vi "TDMS - File Viewer.vi"(4 "error in (no error)":errorcluster, 7 "file path":path) -> (0 "error out":errorcluster, 3 "file path out":path)   [LabVIEW 2017]
doc: "<B>Copyright:</B> (c) 2017 National Instruments. All rights reserved.\n\nOpens the .tdms file specified in the <B>file path</B> input and presents the file data in the TDMS File Viewer dialog box."
uses:
  <vilib>/Utility/tdmsutil.llb/fileViewerConfigData.ctl
  <vilib>/Utility/error.llb/DialogType.ctl
  <vilib>/event_ctls.llb/sizeaction.ctl
  <vilib>/event_ctls.llb/panelstate.ctl
  <vilib>/Utility/tdmsutil.llb/TDMSFileViewerLocalizedText.vi
  Instance           1 26Saved   TDMS - File Viewer .vi
panel:
  out "LastXScaleFormat":u8
  out "TotalCount":u64
  out "Temp Configuration":T1
  in  "LastTopLeftValue":u64
  out "Resize?":bool
  in  "Help":bool
  in  "Status":string
  in  "Quit":bool
  in  "Settings...":bool
  in  "Properties / Values / Graph":T2(tab)
  in  "Properties":i32(listbox)
  in  "Go To":bool
  in  "Scrollbar":u64(c297)
  in  "Raw data values":i32(listbox)
  out "Waveform Graph":waveform(dbl)[](graph)
  in  "File contents":string(tree)
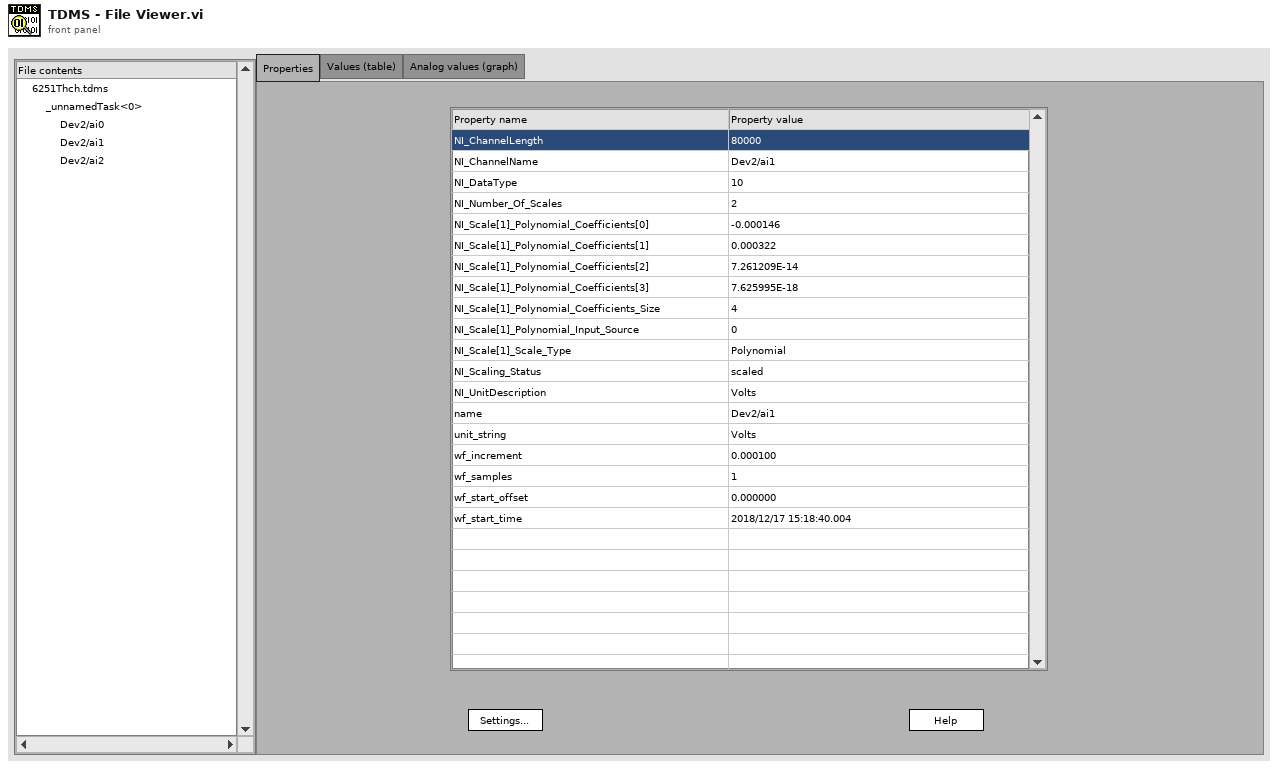
[diagram p1: front panel]
types:
  T1 = typedef "fileViewerConfigData.ctl" = cluster{"Show all (table)":bool, "Show all (graph)":bool, "limit (table)":u64, "limit (graph)":u64, "no show":bool, "start (table)":u64, "start (graph)":u64}
  T2 = enum32{"Properties", "Values (table)", "Analog values (graph)"}
  T3 = enum16{"open", "open or create", "create or replace", "create", "open (read-only)"}
  T4 = cluster{"Tree":refnum<vi>, "Tab Control":refnum<vi>, "property list":refnum<vi>, "raw data list":refnum<vi>, "Waveform Graph":refnum<vi>, "Ok":refnum<vi>, "Ok 2":refnum<vi>, "Ok 3":refnum<vi>, "Ok 4":refnum<vi>, "Scrollbar":refnum<vi>, "Ok 5":refnum<vi>, "TopLeftValue":refnum<vi>, "TotalCount":refnum<vi>}
  T5 = typedef "panelstate.ctl" = enum32{"Standard", "Minimized", "Maximized"}
  T6 = typedef "sizeaction.ctl" = enum32{"Minimized", "Maximized", "Resized"}
  T7 = cluster{"Shift":bool, "Ctrl":bool, "Alt":bool, "Cmd":bool, "Opt":bool}
  T8 = typedef "LVRectTypeDef.ctl" = cluster{"Left":i16, "Top":i16, "Right":i16, "Bottom":i16}
  T9 = typedef "LVRowAndColumnUnsignedTypeDef.ctl" = cluster{"Row":u32, "Column":u32}
  T10 = typedef "DialogType.ctl" = u16
  T11 = typedef "eventvkey.ctl" = enum16{"ASCII", "Enter", "Return", "Shift", "Ctrl", "Alt", "Cmd", "Opt", "Caps", "NumLock", "Clear", "Break", "Up", "Down", "Left", "Right", "Insert", "Delete", "Home", "End", "PageUp", "PageDown", "Escape", "Help", "Pause", "ScrollLock", "F1", "F2", "F3", "F4", "F5", "F6", "F7", "F8", "F9", "F10", "F11", "F12", "F13", "F14", "F15", "F16", "F17", "F18", "F19", "F20", "F21", "F22", "F23", "F24", "Play", "VolumeUp", "VolumeDown", "Mute", "Two Byte Char"}
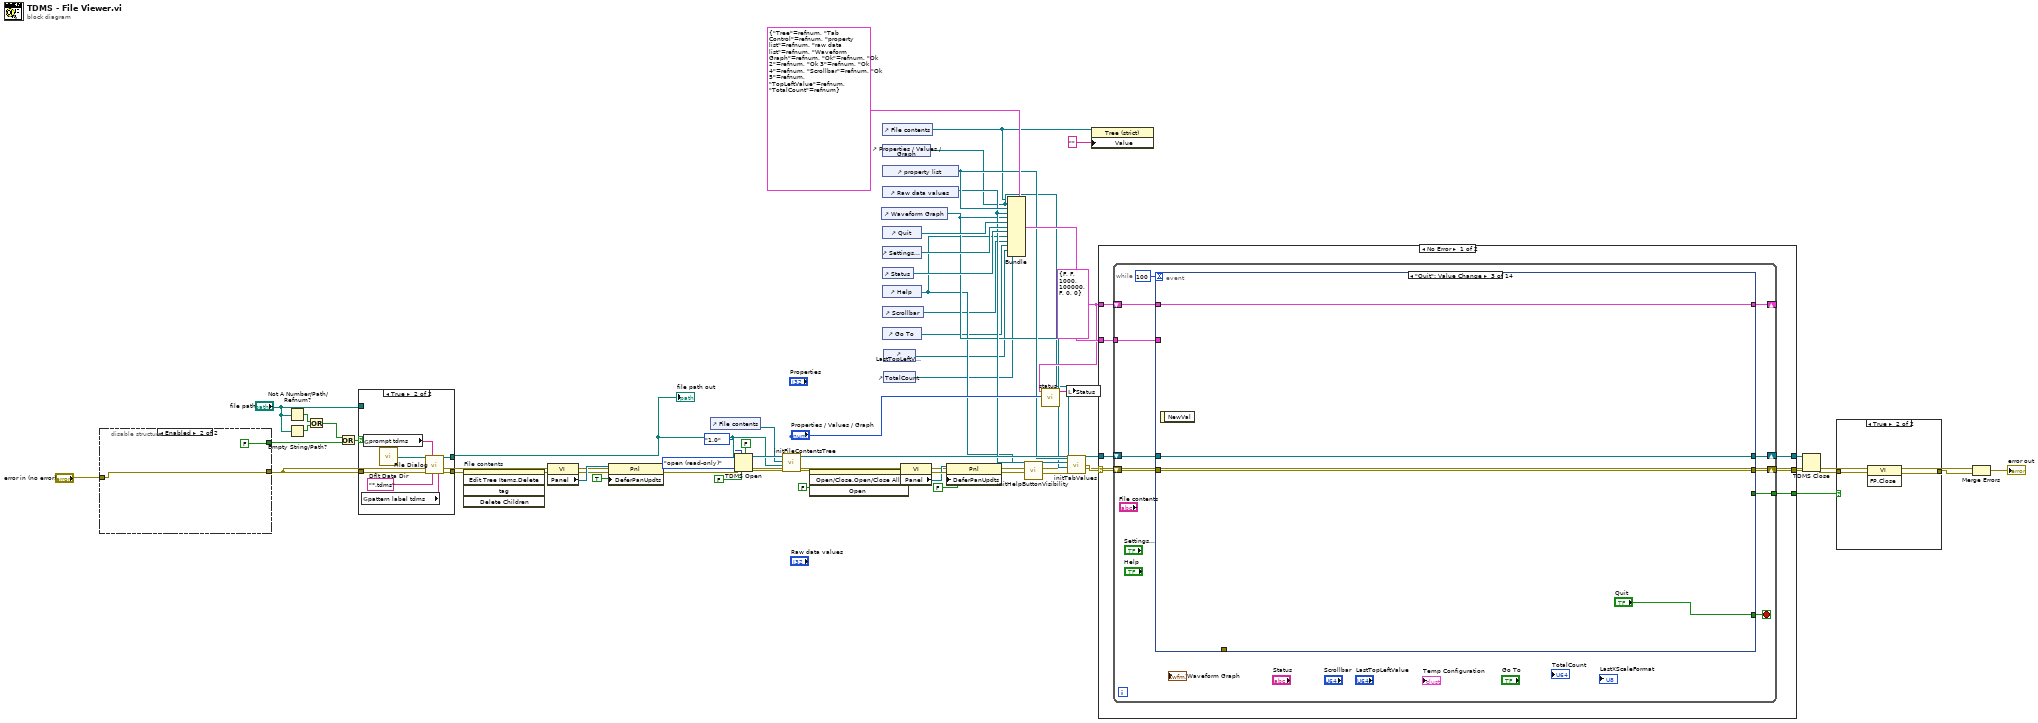
[diagram p0: block diagram]
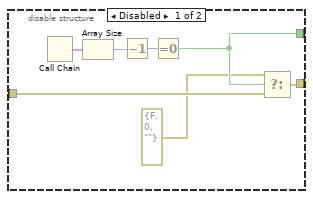
[diagram p2: hidden frame]
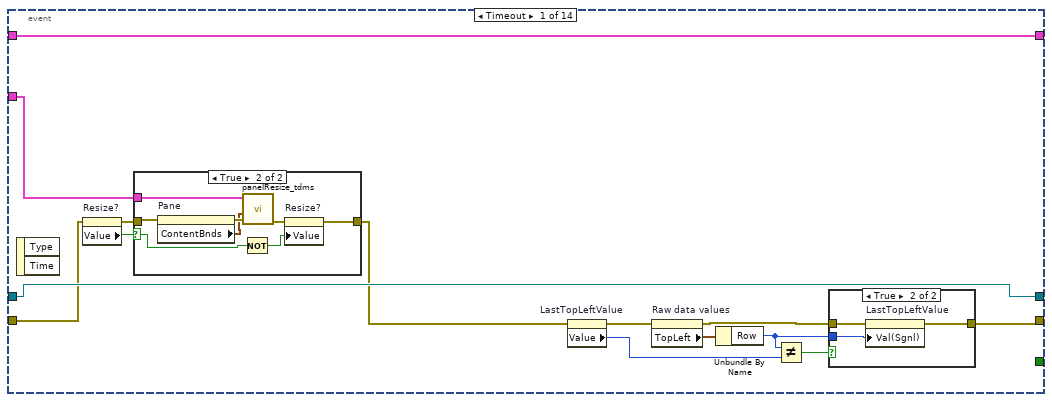
[diagram p4: hidden frame]
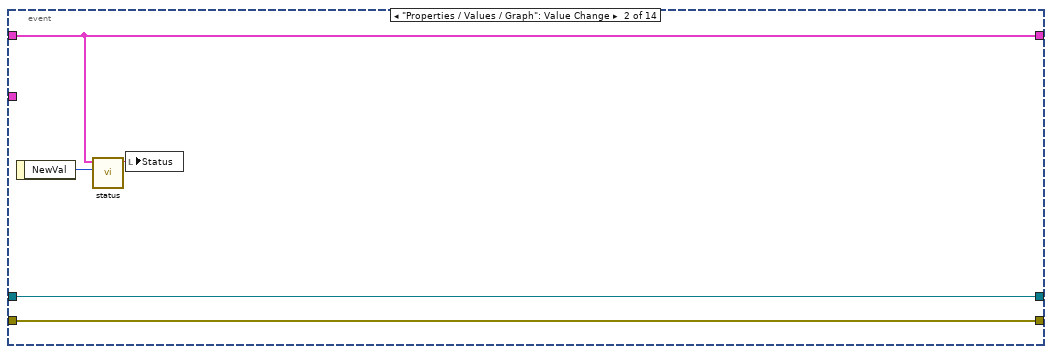
[diagram p7: hidden frame]
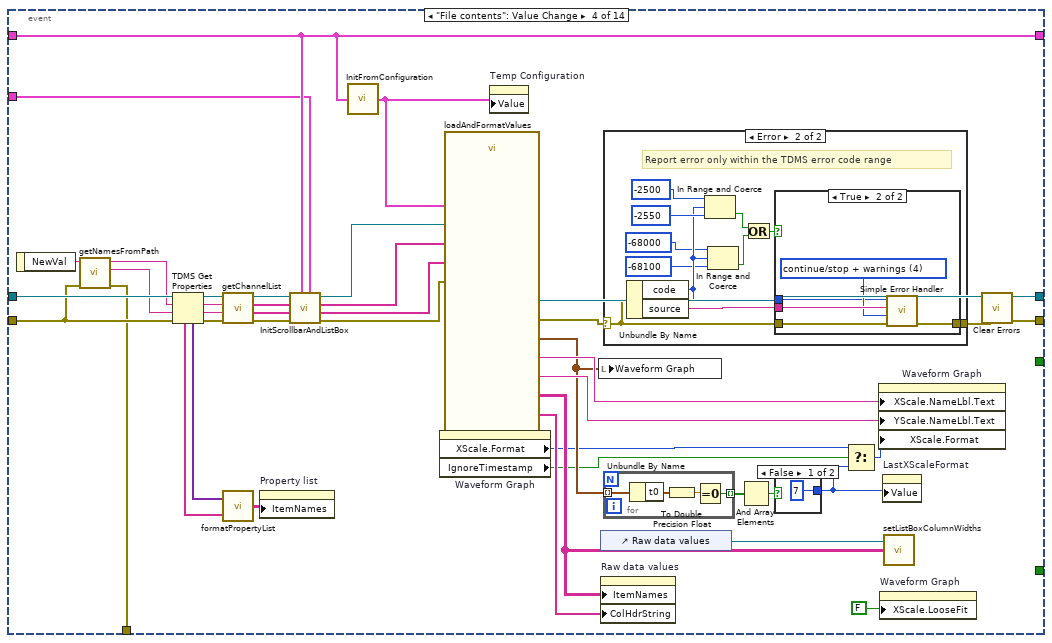
[diagram p8: hidden frame]
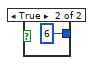
[diagram p9: hidden frame]
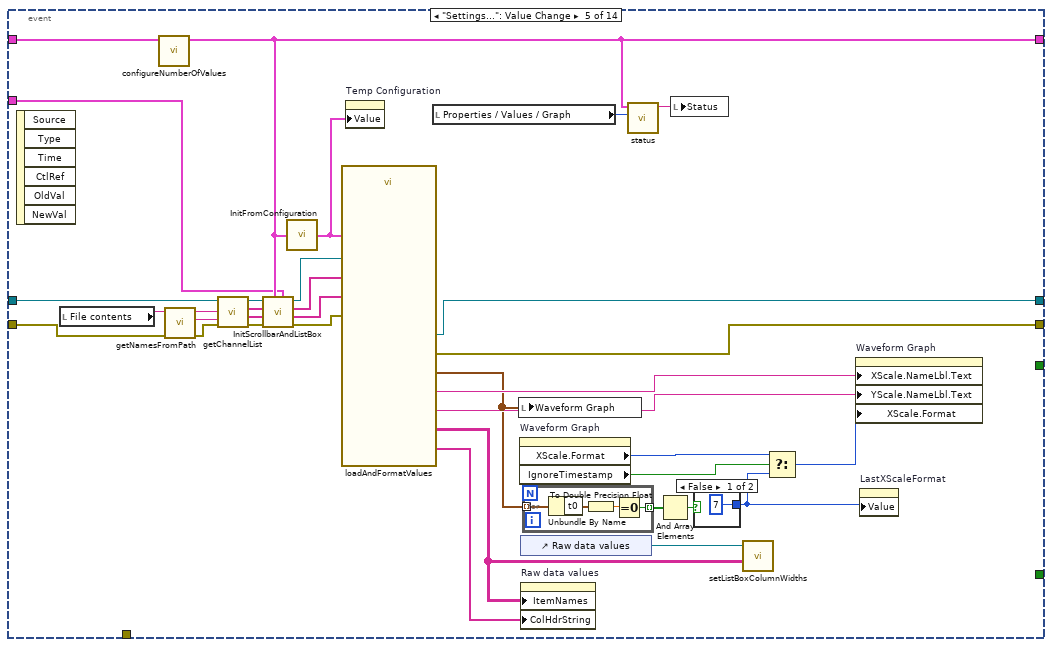
[diagram p12: hidden frame]
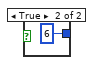
[diagram p13: hidden frame]
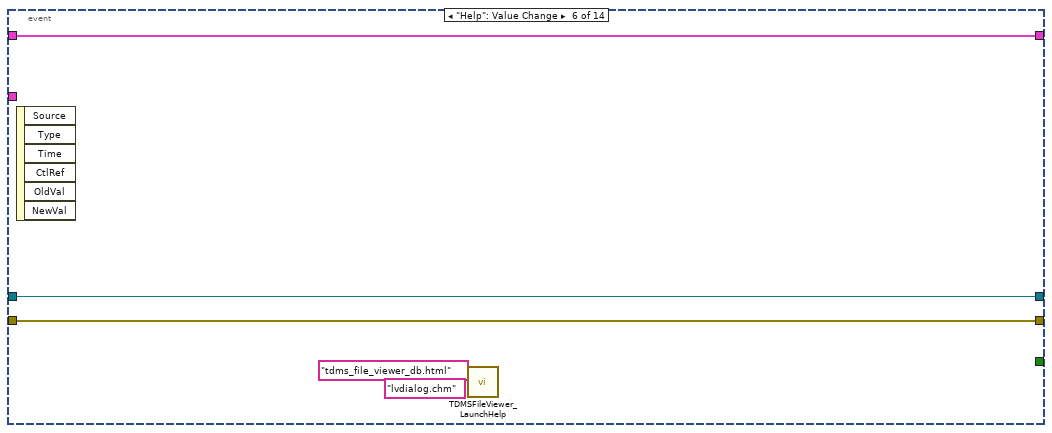
[diagram p14: hidden frame]
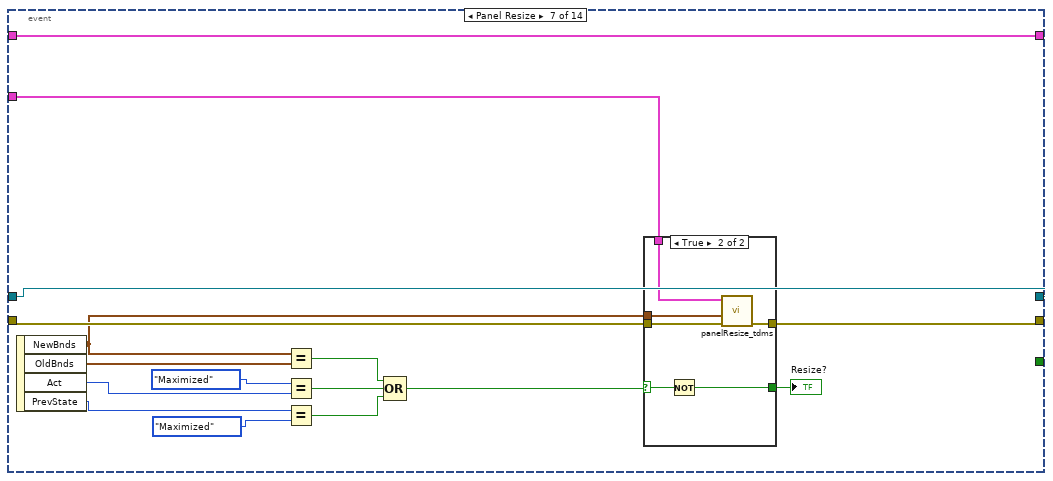
[diagram p15: hidden frame]
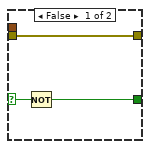
[diagram p16: hidden frame]
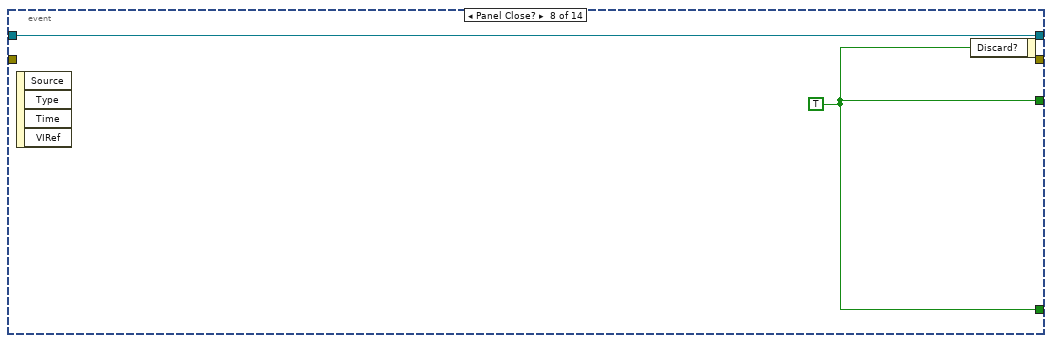
[diagram p17: hidden frame]
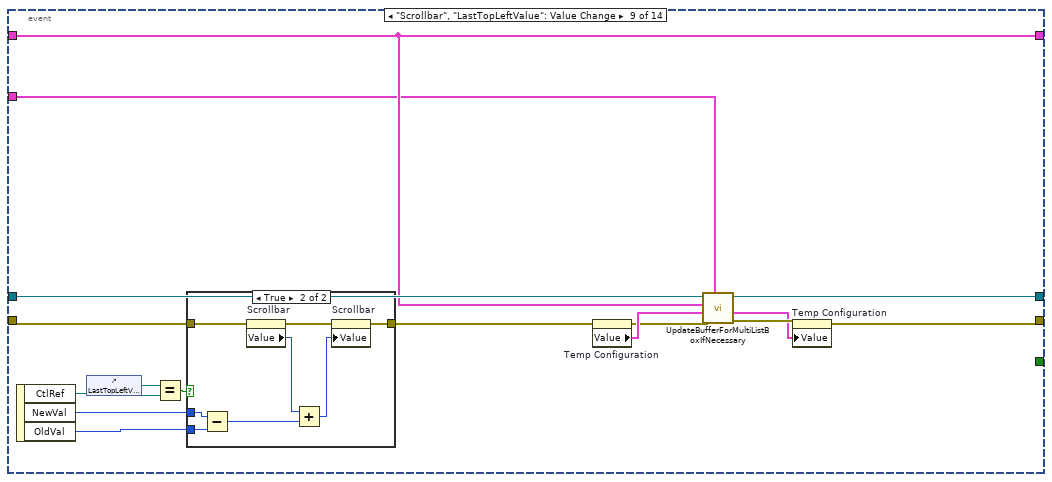
[diagram p18: hidden frame]
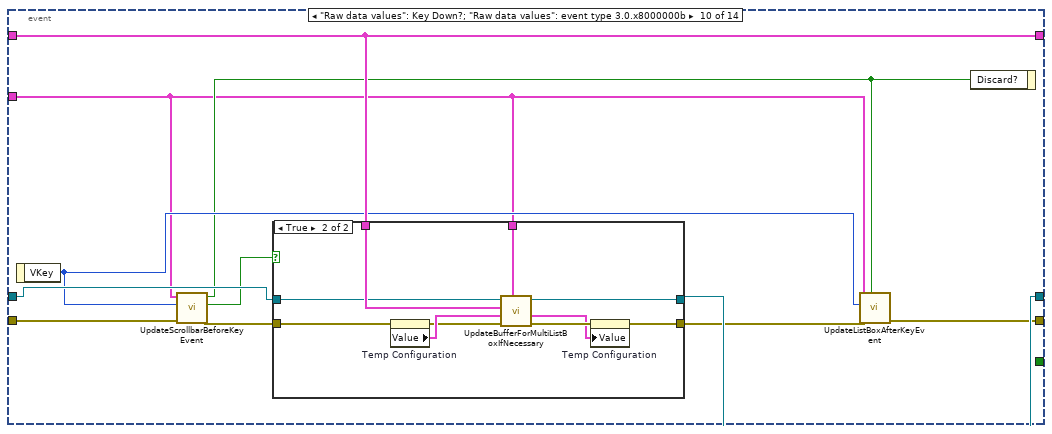
[diagram p20: hidden frame]
diagram:
  w27 = T1 {"Show all (table)"=FALSE, "Show all (graph)"=FALSE, "limit (table)"=1000, "limit (graph)"=100000, "no show"=FALSE, "start (table)"=0, "start (graph)"=0} ("TDMS File Viewer Configuration")
  n1 = disable-structure shown="Enabled" {
    disable-tunnel: [w61 FALSE] -> w25
    disable-tunnel: "error in (no error)" -> [w60 w66]
    disable-tunnel: [w58 w66] -> w7
    frame Disabled {
      n2 = Call Chain() -> (call chain=w64:string[])
      n3 = Array Size(array=w64) -> (size(s)=w63:i32)
      n4 = Decrement(x=w63) -> (x-1=w62:i32)
      n5 = Equal To 0?(x=w62) -> (x = 0?=w61:bool)
      n6 = Select(t=errorcluster {"status"=FALSE, "code"=0, "source"=""}, s=w61, f=w60) -> (s? t:f=w58:errorcluster)
    }
    frame Enabled {
    }
  }
  n7 = Not A Number/Path/Refnum?(number/path/refnum="file path") -> (NaN/Path/Refnum?=w40:bool)
  n8 = Empty String/Path?(string/path="file path") -> (empty?=w39:bool)
  n9 = Or(x=w40, y=w39) -> (x .or. y?=w38:bool)
  n10 = Or(x=w38, y=w25) -> (x .or. y?=w1:bool)
  n11 = case shown="True" w1 {
    tunnel: [w68 w75] -> w31
    tunnel: "file path" -> [w68 _]
    tunnel: [w67 w73] -> w30
    tunnel: w7 -> [w67 w72]
    frame False {
    }
    frame True {
      n12 = global read "TDMSFileViewerLocalizedText.vi" "pattern label tdms"() -> (w70:string)
      n13 = global read "TDMSFileViewerLocalizedText.vi" "prompt tdms"() -> (w71:string)
      n14 = call <vilib>:"Dflt Data Dir.vi"() -> ("App:Default Data Directory"=w69:path)
      n15 = call "File Dialog"("start path"=w69, "prompt"=w71, "error in"=w72, "pattern (all files)"="*.tdms", "pattern label"=w70) -> ("selected path"=w75:path, "error out"=w73:errorcluster)  [unwired: 2 in, 7 out]
    }
  }
  "file path out" <- w31
  n16 = invoke on="File contents" class="Tree (strict)" method="Edit Tree Items.Delete"(error in=w30) -> (error out=w48:errorcluster)  [unwired: 4 in, 4 out]
  n17 = property class="VI"(error in=w48) -> (error out=w49:errorcluster, "Panel"=w50:refnum<vi>)  [unwired: 1 in, 1 out]
  n18 = property class="Pnl"(reference=w50, error in=w49, "DeferPanUpdts"=TRUE ("Defer Panel Updates")) -> (error out=w52:errorcluster)  [unwired: 1 out]
  n19 = control-ref of="File contents"() -> (w32:refnum<vi>)
  n20 = TDMS Open(5:FALSE ("create index file? (T)"), 6:FALSE ("disable buffering (T)"), 7:enum16{"1.0", "2.0"}."1.0" ("file format version (2.0)"), 8:w52, 10:T3."open (read-only)" ("operation"), 11:w31) -> (0:w57:errorcluster, 3:w56:refnum<k34>)  [unwired: 1 in]
  n21 = call <vilib>:"initFileContentsTree.vi"("error in (no error)"=w57, "file path"=w31, "Tree Refnum"=w32, "tdms file"=w56) -> ("error out"=w44:errorcluster, "tdms file out"=w55:refnum<k34>)  [unwired: 2 out]
  n22 = invoke on="File contents" class="Tree (strict)" method="Open/Close.Open/Close All"(error in=w44, "Open"=FALSE ("Open?")) -> (error out=w43:errorcluster)  [unwired: 2 in, 3 out]
  n23 = control-ref of="Waveform Graph"() -> (w16:refnum<vi>)
  n24 = control-ref of="File contents"() -> (w14:refnum<vi>)
  n25 = control-ref of="property list"() -> (w18:refnum<vi>)
  n26 = control-ref of="Raw data values"() -> (w17:refnum<vi>)
  n27 = control-ref of="Quit"() -> (w36:refnum<vi>)
  n28 = control-ref of="Settings..."() -> (w34:refnum<vi>)
  n29 = control-ref of="Help"() -> (w10:refnum<vi>)
  n30 = control-ref of="Scrollbar"() -> (w6:refnum<vi>)
  n31 = control-ref of="Go To"() -> (w5:refnum<vi>)
  n32 = control-ref of="Properties / Values / Graph"() -> (w15:refnum<vi>)
  n33 = control-ref of="Status"() -> (w29:refnum<vi>)
  n34 = control-ref of="LastTopLeftValue"() -> (w4:refnum<vi>)
  n35 = control-ref of="TotalCount"() -> (w3:refnum<vi>)
  n36 = property class="VI"(error in=w43) -> (error out=w46:errorcluster, "Panel"=w45:refnum<vi>)  [unwired: 1 in, 1 out]
  n37 = property class="Pnl"(reference=w45, error in=w46, "DeferPanUpdts"=FALSE ("Defer Panel Updates")) -> (error out=w12:errorcluster)  [unwired: 1 out]
  n38 = Bundle(cluster=T4 {"Tree"=refnum, "Tab Control"=refnum, "property list"=refnum, "raw data list"=refnum, "Waveform Graph"=refnum, "Ok"=refnum, "Ok 2"=refnum, "Ok 3"=refnum, "Ok 4"=refnum, "Scrollbar"=refnum, "Ok 5"=refnum, "TopLeftValue"=refnum, "TotalCount"=refnum} ("control refs"), "Tree"=w14, "Tab Control"=w15, "property list"=w18, "raw data list"=w17, "Waveform Graph"=w16, "Ok"=w36, "Ok 2"=w34, "Ok 3"=w29, "Ok 4"=w10, "Scrollbar"=w6, "Ok 5"=w5, "TopLeftValue"=w4, "TotalCount"=w3) -> (w37:T4)
  n39 = call <vilib>:"initHelpButtonVisibility.vi"("error in"=w12, "Help"=w10) -> ("error out"=w11:errorcluster)  [unwired: 9 in]
  n40 = call <vilib>:"status.vi"("tab sheet"="Properties / Values / Graph", "TDMS File Viewer Configuration"=w27) -> ("status"=w28:string)  [unwired: 5 out]
  n41 = local write "Status"(w28) -> ()
  n42 = call <vilib>:"initTabValues.vi"("properties"=w18, "Values"=w17, "waveform"=w16, "error in"=w11, "Properties / Values / Graph"=w15) -> ("error out"=w19:errorcluster)
  n43 = property class="Tree (strict)"(reference=w14, "Value"="") -> ()  [unwired: 1 in, 2 out]
  n44 = case shown="No Error" w19 {
    selector: w19 -> [w77 w399]
    tunnel: w55 -> [w82 w400]
    tunnel: [w81 w400] -> w54
    tunnel: [w80 w398] -> w53
    tunnel: w37 -> [w79 _]
    tunnel: w27 -> [w78 _]
    tunnel: [w76 FALSE] -> w23
    frame No Error {
      n45 = while {
        shift-right: [w90] -> w80
        shift-left: w77 -> [w91]
        shift-right: [w89] -> w81
        shift-left: w82 -> [w92]
        tunnel: w79 -> [w87]
        shift-right: [w85] -> _
        shift-left: w78 -> [w86]
        tunnel: [w84] -> w76
        stop <- w88 stop-if-true
        n46 = event shown="[2] \"Quit\": Value Change" {
          selector: _ -> [_ _ _ _ _ _ _ _ _ _ _ _ _ _]
          dyn-events: _ -> [_ _ _ _ _ _ _ _ _ _ _ _ _ _]
          timeout: 100 -> [_ _ _ _ _ _ _ _ _ _ _ _ _ _]
          tunnel: w92 -> [w106 w123 w127 w169 w217 w237 w254 w265 w281 w300 w325 w340 w373 w390]
          tunnel: w91 -> [w101 w124 w126 w161 w224 w236 w252 _ w268 w292 w314 w337 w372 w389]
          tunnel: [w94 w124 w126 w157 w225 w236 w251 _ w275 w297 w317 w338 w372 w381] -> w90
          tunnel: [w106 w123 w127 w168 w226 w237 w254 w265 w280 w299 w324 w339 w373 w390] -> w89
          tunnel: [_ _ "Quit" _ _ _ _ w264 _ _ _ _ _ _] -> w88
          tunnel: [_ _ _ w160 _ _ _ _ _ _ _ _ _ _] -> _
          tunnel: w87 -> [w102 _ _ w136 w201 _ w253 _ w267 w293 w315 w334 _ _]
          tunnel: w86 -> [w105 w120 w125 w137 w227 w238 w250 _ w279 w301 w326 w341 w374 w391]
          tunnel: [w105 w120 w125 w137 w203 w238 w250 _ w279 w301 w326 w341 w374 w391] -> w85
          tunnel: [_ _ _ _ _ _ _ w264 _ _ _ _ _ _] -> w84
          event Timeout {
            n47 = event-data() -> ()  [unwired: 3 out]
            n48 = property on="Resize?" class="Bool (strict)"(error in=w101) -> (error out=w103:errorcluster, "Value"=w104:bool)  [unwired: 1 in, 1 out]
            n49 = case shown="True" w104 {
              selector: w104 -> [_ w118]
              tunnel: w102 -> [_ w119]
              tunnel: w103 -> [w111 w114]
              tunnel: [w111 w116] -> w99
              frame False {
              }
              frame True {
                n50 = property on="Pane" class="Pane"(error in=w114) -> (error out=w113:errorcluster, "ContentBnds"=w112:T8)  [unwired: 1 in, 1 out]
                n51 = Not(x=w118) -> (.not. x?=w115:bool)
                n52 = call <vilib>:"panelResize_tdms.vi"("error in (no error)"=w113, "NewBnds"=w112, "control refs"=w119) -> ("error out"=w117:errorcluster)  [unwired: 4 in]
                n53 = property on="Resize?" class="Bool (strict)"(error in=w117, "Value"=w115) -> (error out=w116:errorcluster)  [unwired: 1 in, 1 out]
              }
            }
            n54 = property on="LastTopLeftValue" class="DigNum (strict)"(error in=w99) -> (error out=w98:errorcluster, "Value"=w97:u64)  [unwired: 1 in, 1 out]
            n55 = property on="Raw data values" class="MCListbox (strict)"(error in=w98) -> (error out=w95:errorcluster, "TopLeft"=w100:T9)  [unwired: 1 in, 1 out]
            n56 = Unbundle By Name(w100) -> ("Row"=w93:u32)
            n57 = Not Equal?(x=w93, y=w97) -> (x != y?=w96:bool)
            n58 = case shown="True" w96 {
              tunnel: w95 -> [w107 w110]
              tunnel: [w107 w109] -> w94
              tunnel: w93 -> [_ w108]
              frame False {
              }
              frame True {
                n59 = property on="LastTopLeftValue" class="DigNum (strict)"(error in=w110, "Val(Sgnl)"=w108) -> (error out=w109:errorcluster)  [unwired: 1 in, 1 out]
              }
            }
          }
          event "Properties / Values / Graph": Value Change {
            n60 = event-data() -> ("NewVal"=w122:T2)  [unwired: 1 out]
            n61 = call <vilib>:"status.vi"("tab sheet"=w122, "TDMS File Viewer Configuration"=w120) -> ("status"=w121:string)  [unwired: 5 out]
            n62 = local write "Status"(w121) -> ()
          }
          event "Quit": Value Change {
            n63 = event-data() -> ()  [unwired: 2 out]
          }
          event "File contents": Value Change {
            n64 = event-data() -> ("NewVal"=w163:string)  [unwired: 1 out]
            n65 = call <vilib>:"getNamesFromPath.vi"("error in (no error)"=w161, "tree path"=w163) -> ("error out"=w160:errorcluster, "channel"=w166:string, "group"=w167:string)  [unwired: 3 out]
            n66 = TDMS Get Properties(8:w161, 9:w166, 10:w167, 11:w169) -> (0:w155:errorcluster, 1:w154:string, 2:w150:string, 3:w156:refnum<k34>, 4:w164:variant[], 6:w165:string[])  [unwired: 2 out]
            n67 = call <vilib>:"getChannelList.vi"("error in (no error)"=w155, "channel names"=w154, "group name"=w150, "tdms file"=w156) -> ("error out"=w145:errorcluster, "channel names out"=w143:string[], "group names out"=w141:string[], "tdms file out"=w139:refnum<k34>)
            n68 = call <vilib>:"formatPropertyList.vi"("property names"=w165, "property values"=w164) -> ("strings"=w162:string[][])
            n69 = property on="Property list" class="MCListbox (strict)"("ItemNames"=w162) -> ()  [unwired: 2 in, 2 out]
            n70 = call <vilib>:"InitScrollbarAndListBox.vi"("control refs"=w136, "configuration"=w137, "error in (no error)"=w145, "channel names"=w143, "group names"=w141, "tdms in"=w139) -> ("error out"=w144:errorcluster, "channel out"=w142:string[], "group out"=w140:string[], "tdms out"=w138:refnum<k34>)  [unwired: 2 in]
            n71 = call <vilib>:"InitFromConfiguration.vi"("configuration"=w137) -> ("output cluster"=w146:T1)  [unwired: 4 in]
            n72 = property on="Waveform Graph" class="WFGraph (strict)"() -> ("XScale.Format"=w130:u8, "IgnoreTimestamp"=w129:bool)  [unwired: 2 in, 2 out]
            n73 = call <vilib>:"loadAndFormatValues.vi"("error in (no error)"=w144, "configuration"=w146, "channel names"=w142, "group names"=w140, "tdms file"=w138) -> ("error out"=w149:errorcluster, "graph y names"=w152:string, "graph x names"=w151:string, "tdms file out"=w168:refnum<k34>, "waveform values"=w135:waveform(dbl)[], "table values"=w159:string[][], "table headers"=w153:string[])
            n74 = property on="Temp Configuration" class="Clust (strict)"("Value"=w146) -> ()  [unwired: 2 in, 2 out]
            n75 = local write "Waveform Graph"(w135) -> ()
            n76 = control-ref of="Raw data values"() -> (w158:refnum<vi>)
            n77 = property on="Raw data values" class="MCListbox (strict)"("ItemNames"=w159, "ColHdrString"=w153) -> ()  [unwired: 2 in, 2 out]
            n78 = case shown="Error" w149 {
              selector: w149 -> [w176 w186]
              tunnel: [w176 w185] -> w148
              frame No Error {
              }
              frame Error {
                # "Report error only within the TDMS error code range"
                n79 = Unbundle By Name(w186) -> ("code"=w182:i32, "source"=w187:string)
                n80 = In Range and Coerce(upper limit=-2500, x=w182, lower limit=-2550 ("upper limit")) -> (In Range?=w179:bool)  [unwired: 1 out]
                n81 = In Range and Coerce(upper limit=-68000, x=w182, lower limit=-68100) -> (In Range?=w178:bool)  [unwired: 1 out]
                n82 = Or(x=w179, y=w178) -> (x .or. y?=w177:bool)
                n83 = case shown="True" w177 {
                  tunnel: w187 -> [_ w193]
                  tunnel: w186 -> [w188 w192]
                  tunnel: [w188 w191] -> w185
                  tunnel: w182 -> [_ w189]
                  frame False {
                    # "Out of the range of TDMS\nerror code, we don't report\nthem."
                  }
                  frame True {
                    w190 = T10 4 items=["no dialog", "OK message", "continue or stop message", "OK message + warnings", "continue/stop + warnings"] ("type of dialog (OK msg:1)")
                    n84 = call <vilib>:"Simple Error Handler.vi"("error code (no error:0)"=w189, "error source (\" \")"=w193, "type of dialog (OK msg:1)"=w190, "error in (no error)"=w192) -> ("error out"=w191:errorcluster)  [unwired: 1 in, 4 out]
                  }
                }
              }
            }
            n85 = for {
              tunnel: w135 -> [w175] mode=indexing
              tunnel: [w172] -> w134 mode=indexing
              n86 = Unbundle By Name(w175) -> ("t0"=w174:timestamp)
              n87 = To Double Precision Float(number=w174) -> (double precision float=w173:dbl)
              n88 = Equal To 0?(x=w173) -> (x = 0?=w172:bool)
            }
            n89 = And Array Elements(Boolean array=w134) -> (logical AND=w133:bool)
            n90 = case shown="False" w133 {
              tunnel: [u8 7 u8 6] -> w131
              frame False {
              }
              frame True {
              }
            }
            n91 = Select(t=w130, s=w129, f=w131) -> (s? t:f=w132:u8)
            n92 = property on="Waveform Graph" class="WFGraph (strict)"("XScale.NameLbl.Text"=w151, "YScale.NameLbl.Text"=w152, "XScale.Format"=w132) -> ()  [unwired: 2 in, 2 out]
            n93 = property on="Waveform Graph" class="WFGraph (strict)"("XScale.LooseFit"=FALSE ("X Scale.Loose Fit")) -> ()  [unwired: 2 in, 2 out]
            n94 = property on="LastXScaleFormat" class="DigNum (strict)"("Value"=w131) -> ()  [unwired: 2 in, 2 out]
            n95 = call <vilib>:"setListBoxColumnWidths.vi"("table data"=w159, "MCListbox Refnum"=w158) -> ()  [unwired: 1 out]
            n96 = call <vilib>:"Clear Errors.vi"("error in (no error)"=w148) -> ("error out"=w157:errorcluster)  [unwired: 1 in, 5 out]
          }
          event "Settings...": Value Change {
            n97 = event-data() -> ()  [unwired: 7 out]
            n98 = local read "File contents"() -> (w218:string)
            n99 = call <vilib>:"configureNumberOfValues.vi"("TDMS File Viewer Configuration"=w227) -> ("TDMS File Viewer Configuration Out"=w203:T1)  [unwired: 10 out]
            n100 = call <vilib>:"getNamesFromPath.vi"("error in (no error)"=w224, "tree path"=w218) -> ("error out"=w216:errorcluster, "channel"=w214:string, "group"=w215:string)  [unwired: 3 out]
            n101 = call <vilib>:"getChannelList.vi"("error in (no error)"=w216, "channel names"=w214, "group name"=w215, "tdms file"=w217) -> ("error out"=w205:errorcluster, "channel names out"=w207:string[], "group names out"=w209:string[], "tdms file out"=w211:refnum<k34>)
            n102 = call <vilib>:"InitScrollbarAndListBox.vi"("control refs"=w201, "configuration"=w203, "error in (no error)"=w205, "channel names"=w207, "group names"=w209, "tdms in"=w211) -> ("error out"=w204:errorcluster, "channel out"=w206:string[], "group out"=w208:string[], "tdms out"=w210:refnum<k34>)  [unwired: 2 in]
            n103 = call <vilib>:"InitFromConfiguration.vi"("configuration"=w203) -> ("output cluster"=w202:T1)  [unwired: 4 in]
            n104 = call <vilib>:"loadAndFormatValues.vi"("error in (no error)"=w204, "configuration"=w202, "channel names"=w206, "group names"=w208, "tdms file"=w210) -> ("error out"=w225:errorcluster, "graph y names"=w220:string, "graph x names"=w219:string, "tdms file out"=w226:refnum<k34>, "waveform values"=w198:waveform(dbl)[], "table values"=w221:string[][], "table headers"=w223:string[])
            n105 = property on="Temp Configuration" class="Clust (strict)"("Value"=w202) -> ()  [unwired: 2 in, 2 out]
            n106 = local read "Properties / Values / Graph"() -> (w212:T2)
            n107 = local write "Waveform Graph"(w198) -> ()
            n108 = property on="Waveform Graph" class="WFGraph (strict)"() -> ("XScale.Format"=w195:u8, "IgnoreTimestamp"=w194:bool)  [unwired: 2 in, 2 out]
            n109 = control-ref of="Raw data values"() -> (w222:refnum<vi>)
            n110 = property on="Raw data values" class="MCListbox (strict)"("ItemNames"=w221, "ColHdrString"=w223) -> ()  [unwired: 2 in, 2 out]
            n111 = for {
              tunnel: w198 -> [w233] mode=indexing
              tunnel: [w230] -> w200 mode=indexing
              n112 = Unbundle By Name(w233) -> ("t0"=w232:timestamp)
              n113 = To Double Precision Float(number=w232) -> (double precision float=w231:dbl)
              n114 = Equal To 0?(x=w231) -> (x = 0?=w230:bool)
            }
            n115 = call <vilib>:"status.vi"("tab sheet"=w212, "TDMS File Viewer Configuration"=w203) -> ("status"=w213:string)  [unwired: 5 out]
            n116 = And Array Elements(Boolean array=w200) -> (logical AND=w199:bool)
            n117 = local write "Status"(w213) -> ()
            n118 = case shown="False" w199 {
              tunnel: [u8 7 u8 6] -> w196
              frame False {
              }
              frame True {
              }
            }
            n119 = call <vilib>:"setListBoxColumnWidths.vi"("table data"=w221, "MCListbox Refnum"=w222) -> ()  [unwired: 1 out]
            n120 = Select(t=w195, s=w194, f=w196) -> (s? t:f=w197:u8)
            n121 = property on="Waveform Graph" class="WFGraph (strict)"("XScale.NameLbl.Text"=w219, "YScale.NameLbl.Text"=w220, "XScale.Format"=w197) -> ()  [unwired: 2 in, 2 out]
            n122 = property on="LastXScaleFormat" class="DigNum (strict)"("Value"=w196) -> ()  [unwired: 2 in, 2 out]
          }
          event "Help": Value Change {
            n123 = event-data() -> ()  [unwired: 7 out]
            n124 = call <vilib>:"TDMSFileViewer_LaunchHelp.vi"("CHM or HLP filename (lvdialog.chm)"="lvdialog.chm", "HTML filename"="tdms_file_viewer_db.html") -> ()  [unwired: 1 in, 5 out]
          }
          event Panel Resize {
            n125 = event-data() -> ("NewBnds"=w242:T8, "OldBnds"=w241:T8, "Act"=w243:T6, "PrevState"=w244:T5)  [unwired: 1 out]
            n126 = Equal?(x=w242, y=w241) -> (x = y?=w247:bool)
            n127 = Equal?(x=sizeaction."Maximized" ("Act"), y=w243) -> (x = y?=w246:bool)
            n128 = Equal?(x=w244, y=panelstate."Maximized" ("PrevState")) -> (x = y?=w245:bool)
            n129 = Compound Arithmetic op=OR(w247, w246, w245) -> (w240:bool)
            n130 = case shown="True" w240 {
              selector: w240 -> [w256 w259]
              tunnel: w253 -> [_ w263]
              tunnel: w252 -> [w257 w262]
              tunnel: [w257 w261] -> w251
              tunnel: w242 -> [_ w260]
              tunnel: [w255 w258] -> w239
              frame False {
                n131 = Not(x=w256) -> (.not. x?=w255:bool)
              }
              frame True {
                n132 = Not(x=w259) -> (.not. x?=w258:bool)
                n133 = call <vilib>:"panelResize_tdms.vi"("error in (no error)"=w262, "NewBnds"=w260, "control refs"=w263) -> ("error out"=w261:errorcluster)  [unwired: 4 in]
              }
            }
            "Resize?" <- w239
          }
          event Panel Close? {
            w264 = TRUE
            n134 = event-data() -> ()  [unwired: 5 out]
            n135 = event-data("Discard?"=w264) -> ()  [unwired: 1 in, 1 out]
          }
          event "Scrollbar", "LastTopLeftValue": Value Change {
            n136 = event-data() -> ("CtlRef"=w273:refnum<vi>, "NewVal"=w270:u64, "OldVal"=w269:u64)  [unwired: 1 out]
            n137 = control-ref of="LastTopLeftValue"() -> (w272:refnum<vi>)
            n138 = Equal?(x=w272, y=w273) -> (x = y?=w271:bool)
            n139 = case shown="True" w271 {
              tunnel: w270 -> [_ w286]
              tunnel: w269 -> [_ w285]
              tunnel: w268 -> [w282 w284]
              tunnel: [w282 w283] -> w266
              frame False {
              }
              frame True {
                n140 = Subtract(x=w286, y=w285) -> (x-y=w288:u64)
                n141 = property on="Scrollbar" class="Scroll (strict)"(error in=w284) -> (error out=w290:errorcluster, "Value"=w289:u64)  [unwired: 1 in, 1 out]
                n142 = Add(x=w289, y=w288) -> (x+y=w287:u64)
                n143 = property on="Scrollbar" class="Scroll (strict)"(error in=w290, "Value"=w287) -> (error out=w283:errorcluster)  [unwired: 1 in, 1 out]
              }
            }
            n144 = property on="Temp Configuration" class="Clust (strict)"(error in=w266) -> (error out=w277:errorcluster, "Value"=w278:T1)  [unwired: 1 in, 1 out]
            n145 = call <vilib>:"UpdateBufferForMultiListBoxIfNecessary.vi"("control refs"=w267, "error in"=w277, "Buffer Configuration"=w278, "TDMS File Viewer Configuration"=w279, "tdms file in"=w281) -> ("error out"=w276:errorcluster, "BufferConfig out"=w274:T1, "tdms file out"=w280:refnum<k34>)  [unwired: 4 in]
            n146 = property on="Temp Configuration" class="Clust (strict)"(error in=w276, "Value"=w274) -> (error out=w275:errorcluster)  [unwired: 1 in, 1 out]
          }
          event "Raw data values": Key Down?; "Raw data values": event type 3.0.x8000000b {
            n147 = event-data() -> ("VKey"=w295:T11)  [unwired: 1 out]
            n148 = call <vilib>:"UpdateScrollbarBeforeKeyEvent.vi"("error in (no error)"=w292, "VKey"=w295, "control refs 2"=w293) -> ("error out"=w298:errorcluster, "LoadBuffer?"=w296:bool, "DiscardEvent?"=w294:bool)  [unwired: 6 in]
            n149 = case shown="True" w296 {
              tunnel: w301 -> [_ w309]
              tunnel: w300 -> [w302 w308]
              tunnel: [w302 w307] -> w299
              tunnel: w298 -> [w303 w304]
              tunnel: [w303 w306] -> w291
              tunnel: w293 -> [_ w305]
              frame False {
              }
              frame True {
                n150 = property on="Temp Configuration" class="Clust (strict)"(error in=w304) -> (error out=w312:errorcluster, "Value"=w313:T1)  [unwired: 1 in, 1 out]
                n151 = call <vilib>:"UpdateBufferForMultiListBoxIfNecessary.vi"("control refs"=w305, "error in"=w312, "Buffer Configuration"=w313, "TDMS File Viewer Configuration"=w309, "tdms file in"=w308) -> ("error out"=w311:errorcluster, "BufferConfig out"=w310:T1, "tdms file out"=w307:refnum<k34>)  [unwired: 4 in]
                n152 = property on="Temp Configuration" class="Clust (strict)"(error in=w311, "Value"=w310) -> (error out=w306:errorcluster)  [unwired: 1 in, 1 out]
              }
            }
            n153 = call <vilib>:"UpdateListBoxAfterKeyEvent.vi"("DiscardEvent?"=w294, "error in (no error)"=w291, "VKey"=w295, "control refs"=w293) -> ("error out"=w297:errorcluster)  [unwired: 7 in]
            n154 = event-data("Discard?"=w294) -> ()  [unwired: 1 in, 1 out]
          }
          event "Go To": Value Change {
            n155 = event-data() -> ()  [unwired: 2 out]
            n156 = call <vilib>:"GoTo.vi"("error in"=w314, "control refs"=w315) -> ("error out"=w323:errorcluster, "VisibleValue"=w320:u64)  [unwired: 8 in]
            n157 = property on="Temp Configuration" class="Clust (strict)"(error in=w323) -> (error out=w329:errorcluster, "Value"=w330:T1)  [unwired: 1 in, 1 out]
            n158 = call <vilib>:"UpdateBufferForMultiListBoxIfNecessary.vi"("control refs"=w315, "error in"=w329, "Buffer Configuration"=w330, "TDMS File Viewer Configuration"=w326, "tdms file in"=w325) -> ("error out"=w328:errorcluster, "BufferConfig out"=w327:T1, "tdms file out"=w324:refnum<k34>)  [unwired: 4 in]
            n159 = property on="Temp Configuration" class="Clust (strict)"(error in=w328, "Value"=w327) -> (error out=w316:errorcluster)  [unwired: 1 in, 1 out]
            n160 = property on="Raw data values" class="MCListbox (strict)"(error in=w316) -> (error out=w318:errorcluster, "TopLeft"=w322:T9)  [unwired: 1 in, 1 out]
            n161 = Unbundle By Name(w322) -> ("Row"=w321:u32)
            n162 = Add(x=w321, y=w320) -> (x+y=w319:u64)
            n163 = property on="Raw data values" class="MCListbox (strict)"(error in=w318, "Value"=w319) -> (error out=w317:errorcluster)  [unwired: 1 in, 1 out]
          }
          event Key Down {
            n164 = event-data() -> ("PlatMods"=w333:T7, "Char"=w332:i16)  [unwired: 1 out]
            n165 = property on="Raw data values" class="MCListbox (strict)"(error in=w337) -> (error out=w331:errorcluster, "Key Focus"=w336:bool)  [unwired: 1 in, 1 out]
            n166 = case shown="True" w336 {
              selector: w336 -> [w342 _]
              tunnel: [w342 w343] -> w335
              tunnel: w333 -> [_ w348]
              tunnel: w332 -> [_ w347]
              frame False {
              }
              frame True {
                n167 = disable-structure shown="Default" {
                  disable-tunnel: [T7 {"Shift"=FALSE, "Ctrl"=TRUE, "Alt"=FALSE, "Cmd"=FALSE, "Opt"=TRUE} ("PlatMods") T7 {"Shift"=FALSE, "Ctrl"=FALSE, "Alt"=FALSE, "Cmd"=TRUE, "Opt"=FALSE} ("PlatMods")] -> w349
                  frame condition #0 (active) {
                  }
                  frame condition #1 {
                  }
                }
                n168 = Equal?(x=w349, y=w348) -> (x = y?=w345:bool)
                n169 = Equal?(x=w347, y=i16 103 ("Char")) -> (x = y?=w344:bool)
                n170 = And(x=w345, y=w344) -> (x .and. y?=w343:bool)
              }
            }
            n171 = case shown="True" w335 {
              tunnel: w341 -> [_ w367]
              tunnel: w340 -> [w352 w366]
              tunnel: [w352 w365] -> w339
              tunnel: [w353 w358] -> w338
              tunnel: w331 -> [w353 w354]
              tunnel: w334 -> [_ w356]
              tunnel: w334 -> [_ w355]
              frame False {
              }
              frame True {
                n172 = call <vilib>:"GoTo.vi"("error in"=w354, "control refs"=w355) -> ("error out"=w364:errorcluster, "VisibleValue"=w361:u64)  [unwired: 8 in]
                n173 = property on="Temp Configuration" class="Clust (strict)"(error in=w364) -> (error out=w370:errorcluster, "Value"=w371:T1)  [unwired: 1 in, 1 out]
                n174 = call <vilib>:"UpdateBufferForMultiListBoxIfNecessary.vi"("control refs"=w356, "error in"=w370, "Buffer Configuration"=w371, "TDMS File Viewer Configuration"=w367, "tdms file in"=w366) -> ("error out"=w369:errorcluster, "BufferConfig out"=w368:T1, "tdms file out"=w365:refnum<k34>)  [unwired: 4 in]
                n175 = property on="Temp Configuration" class="Clust (strict)"(error in=w369, "Value"=w368) -> (error out=w357:errorcluster)  [unwired: 1 in, 1 out]
                n176 = property on="Raw data values" class="MCListbox (strict)"(error in=w357) -> (error out=w359:errorcluster, "TopLeft"=w363:T9)  [unwired: 1 in, 1 out]
                n177 = Unbundle By Name(w363) -> ("Row"=w362:u32)
                n178 = Add(x=w362, y=w361) -> (x+y=w360:u64)
                n179 = property on="Raw data values" class="MCListbox (strict)"(error in=w359, "Value"=w360) -> (error out=w358:errorcluster)  [unwired: 1 in, 1 out]
              }
            }
          }
          event Key Down? {
            n180 = event-data() -> ("VKey"=w376:T11)  [unwired: 1 out]
            n181 = case shown="\"F1\"" w376 {
              tunnel: [FALSE ("Discard?") TRUE ("Discard?")] -> w375
              frame Default {
              }
              frame "F1" {
                n182 = call <vilib>:"TDMSFileViewer_LaunchHelp.vi"("CHM or HLP filename (lvdialog.chm)"="lvdialog.chm", "HTML filename"="tdms_file_viewer_db.html") -> ()  [unwired: 1 in, 5 out]
              }
            }
            n183 = event-data("Discard?"=w375) -> ()  [unwired: 1 in, 1 out]
          }
          event "Waveform Graph": Shortcut Menu Selection (App) {
            n184 = event-data() -> ("ItemTag"=w387:string)  [unwired: 1 out]
            n185 = property on="Waveform Graph" class="WFGraph (strict)"(error in=w389) -> (error out=w382:errorcluster, "IgnoreTimestamp"=w386:bool)  [unwired: 1 in, 1 out]
            n186 = Not(x=w386) -> (.not. x?=w383:bool)
            n187 = Equal?(x=w387, y="APP_SC_IGNORE_TIME_STAMP") -> (x = y?=w384:bool)
            n188 = And(x=w383, y=w384) -> (x .and. y?=w385:bool)
            n189 = case shown="True" w385 {
              tunnel: w382 -> [w392 w396]
              tunnel: [w392 w393] -> w381
              frame False {
              }
              frame True {
                n190 = property on="LastXScaleFormat" class="DigNum (strict)"(error in=w396) -> (error out=w395:errorcluster, "Value"=w394:u8)  [unwired: 1 in, 1 out]
                n191 = property on="Waveform Graph" class="WFGraph (strict)"(error in=w395, "XScale.Format"=w394) -> (error out=w393:errorcluster)  [unwired: 1 in, 1 out]
              }
            }
          }
        }
      }
    }
    frame Error {
      n192 = call <vilib>:"Simple Error Handler.vi"("error in (no error)"=w399) -> ("error out"=w398:errorcluster)  [unwired: 1 in, 7 out]
    }
  }
  n193 = TDMS Close(8:w53, 11:w54) -> (0:w22:errorcluster)  [unwired: 1 out]
  n194 = case shown="True" w23 {
    tunnel: w22 -> [w401 w403]
    tunnel: [w401 w402] -> w9
    frame False {
    }
    frame True {
      n195 = invoke class="VI" method="FP.Close"(error in=w403) -> (error out=w402:errorcluster)  [unwired: 2 in, 2 out]
    }
  }
  n196 = Merge Errors(w7, w9) -> (→"error out":errorcluster)
